vi "Control-Actuator.vi"(0 "DAQ Device IN":T2={"DAQ Fs (S/s)"=10000.0, "task"="", "error"={"status"=FALSE, "code"=0, "source"=""}, "Min Value"=-10.0, "Max Value"=10.0}, 1 "Camera Device  IN":T1, 2 "Image Device IN":cluster{"Image":T4, "errorImage":errorcluster}, 4 "Time Control Parameters":cluster{"# samples":u32, "tiempos (ms)":dbl}, 5 "Limites":T3, 6 "DAQ?":bool, 7 "ControlSignal":dbl[](array[numeric]), 8 "Streeam?":bool) -> (13 "Contraste":dbl, 14 "DAQ Device OUT":T2={"DAQ Fs (S/s)"=0.0, "task"="", "error"={"status"=FALSE, "code"=0, "source"=""}, "Min Value"=-10.0, "Max Value"=10.0}, 15 "Camera Device OUT":T1, 16 "Image Device OUT":cluster{"Image":T4, "errorImage":errorcluster}, 17 "Waveform":waveform(dbl))   [LabVIEW 2010]
uses:
  <vilib>/vision/Image Controls.llb/IMAQ Image.ctl
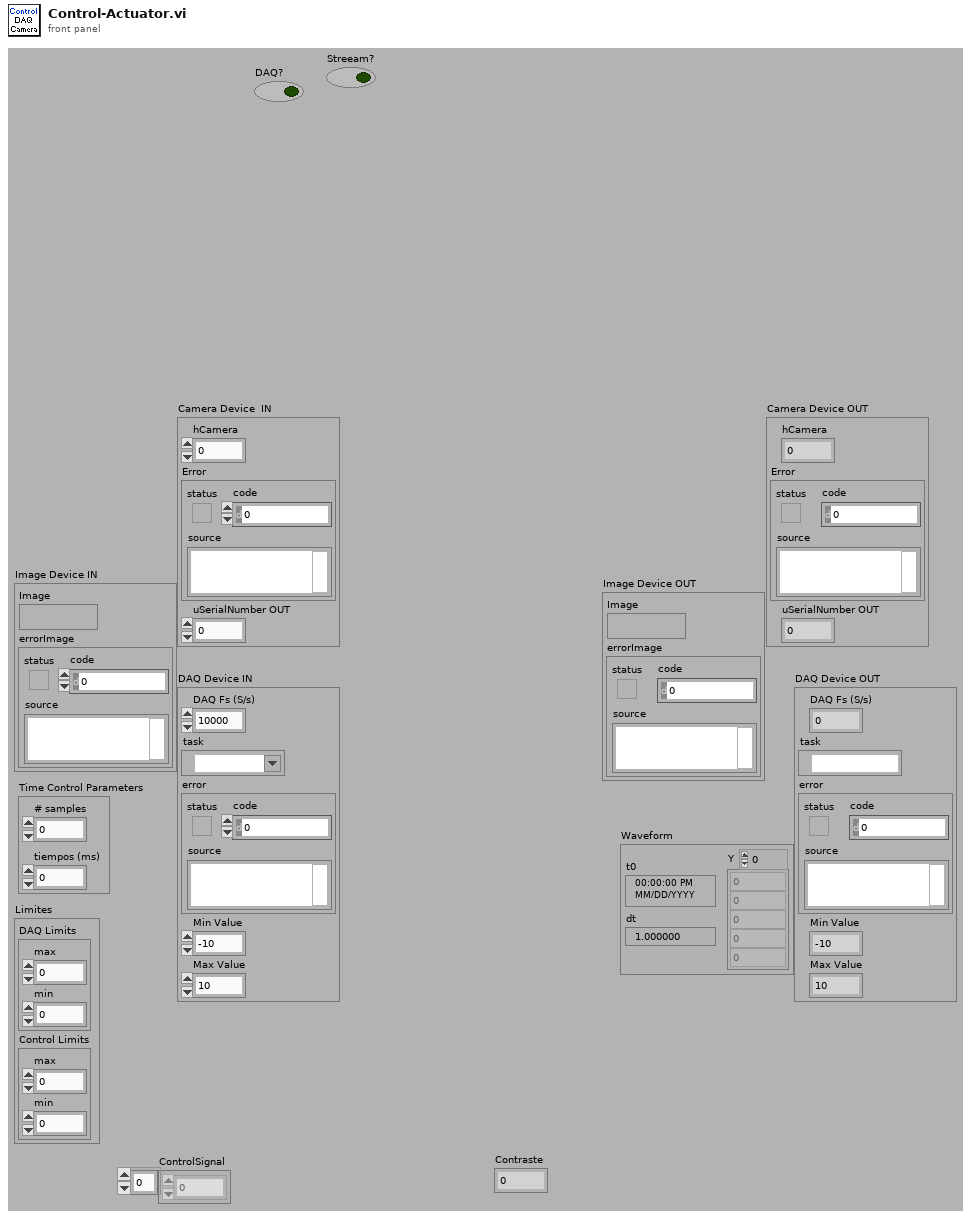
[diagram p1: front panel]
types:
  T1 = cluster{"hCamera":u32, "Error":errorcluster, "uSerialNumber OUT":u32}
  T2 = cluster{"DAQ Fs (S/s)":dbl, "task":refnum<k21>, "error":errorcluster, "Min Value":dbl, "Max Value":dbl}
  T3 = cluster{"DAQ Limits":cluster{"max":dbl, "min":dbl}, "Control Limits":cluster{"max":dbl, "min":dbl}}
  T4 = typedef "IMAQ Image.ctl" = refnum<image>
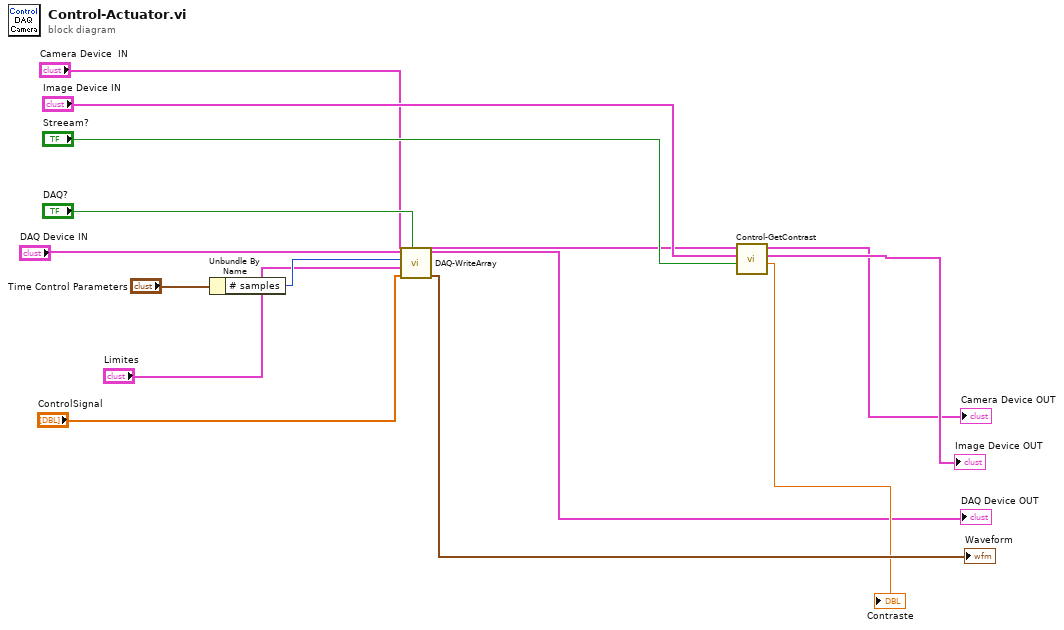
[diagram p0: block diagram]
diagram:
  n1 = Unbundle By Name("Time Control Parameters") -> ("# samples"=w6:u32)
  n2 = call "DAQ-WriteArray.vi"("DAQ?"="DAQ?", "Control Array"="ControlSignal", "Limites"="Limites", "#samples"=w6, "DAQ Device IN"="DAQ Device IN") -> ("Waveform Graph"=→"Waveform":waveform(dbl), "DAQ Device OUT"=→"DAQ Device OUT":T2)  [unwired: 2 in]
  n3 = call "Control-GetContrast.vi"("Streeam?"="Streeam?", "Image Device IN"="Image Device IN", "Camera Device  IN"="Camera Device  IN") -> ("Contraste OUT"=→"Contraste":dbl, "Image Device OUT"=→"Image Device OUT":cluster{"Image":T4, "errorImage":errorcluster}, "Camera Device OUT"=→"Camera Device OUT":T1)  [unwired: 2 in]
